vi "Initialize Experiment File.vi"(8 "error in (no error)":errorcluster, 9 "Experiment File Extension":string, 10 "Experiment Directory":path, 11 "Experiment Name":string) -> (0 "error out":errorcluster, 1 "cancelled":bool, 2 "Experiment Directory out":path, 3 "Experiment Filename out":string, 5 "Experiment File Cluster":T1)   [LabVIEW 2020, in "Experiment File.lvlib"]
doc: "Creates a new default experiment file at the given Experiment Directory using the Experiment Name as the file name, based on the Experiment File.ctl cluster. If the file already exists, it will ask the user if they want to overwrite it or not, where cancelled becomes True if the user declines to overwrite the file or False if they chose to overwrite it."
uses:
  Experiment File.lvlib
  Experiment File Cluster.ctl
  Plugin Servers/Controller/Minimal Controller Cluster.ctl
  Plugin Servers/Parameter to Hardware Map/Minimal Map.ctl
  Plugin Servers/Parameter to Hardware Map/Minimal Pair Cluster.ctl
  Plugin Servers/Controller/Generic Plugin.lvclass
  Plugin Servers/Parameter to Hardware Map/Parameter to Hardware Map.lvclass
panel:
  out "JSON String":string
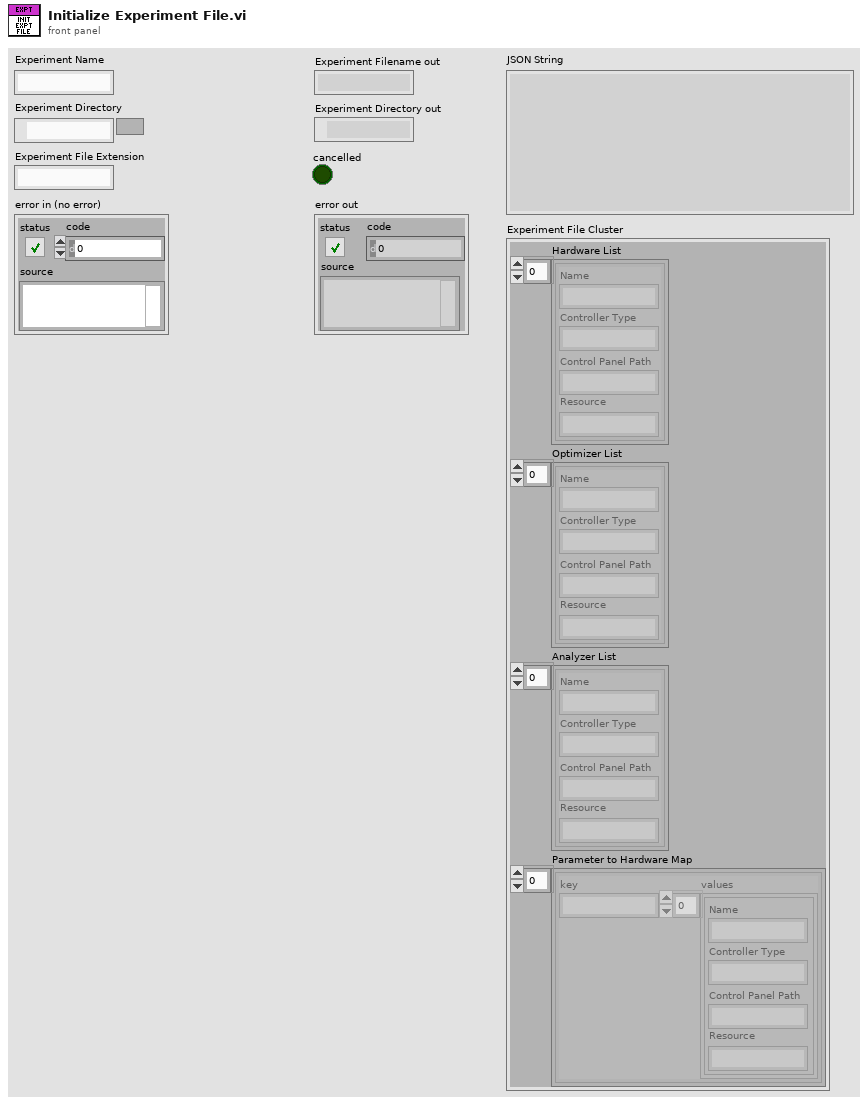
[diagram p1: front panel]
types:
  T1 = typedef "Experiment File.lvlib/Experiment File Cluster.ctl" = cluster{"Hardware List":T2[], "Optimizer List":T2[], "Analyzer List":T2[], "Parameter to Hardware Map":T3}
  T2 = typedef "Generic Plugin.lvclass/Minimal Controller Cluster.ctl" = cluster{"Name":string, "Controller Type":string, "Control Panel Path":string, "Resource":string}
  T3 = typedef "Parameter to Hardware Map.lvclass/Minimal Map.ctl" = T4[]
  T4 = typedef "Parameter to Hardware Map.lvclass/Minimal Pair Cluster.ctl" = cluster{"key":string, "values":T2[]}
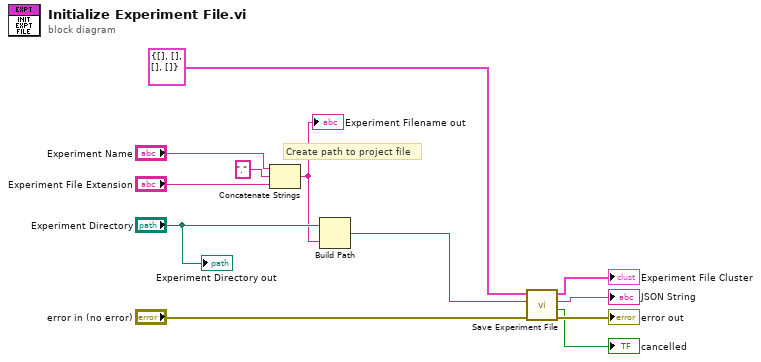
[diagram p0: block diagram]
diagram:
  # "Create path to project file"
  n1 = Concatenate Strings("Experiment Name", "." ("string"), "Experiment File Extension") -> (w10:string)
  "Experiment Filename out" <- w10
  n2 = Build Path(base path="Experiment Directory", name or relative path=w10) -> (appended path=w8:path)
  n3 = call "Save Experiment File.vi"("error in (no error)"="error in (no error)", "Experiment File Full Path"=w8, "Experiment File Cluster"=T1 {"Hardware List"=[], "Optimizer List"=[], "Analyzer List"=[], "Parameter to Hardware Map"=[]} ("File")) -> ("error out"=→"error out":errorcluster, "cancelled"=→"cancelled":bool, "JSON string"=→"JSON String":string, "Experiment File Cluster (duplicate)"=→"Experiment File Cluster":T1)  [unwired: 5 in]
  "Experiment Directory out" <- "Experiment Directory"
